vi "Write REF Channels.vi"(8 "error in (no error)":errorcluster, 10 "REF Channels":T1 {"Roll-Off" min=1; "TC" min=0.0001 format="%#_3p"; "Phase" format="%.3g"; "Frequency" min=0.0001 max=10000.0 format="%.3g"; "Channel" min=1}, 11 "DSP in":refnum<class "DSP.lvclass">) -> (0 "error out":errorcluster, 3 "DSP out":refnum<class "DSP.lvclass">)   [LabVIEW 2019, in "DSP.lvclass"]
uses:
  DSP.lvclass
  DSP.lvclass/DSP.ctl
  Typedefs/REF.Channel--Cluster.ctl
  Typedefs/REF.Channel--Cluster--Array.ctl
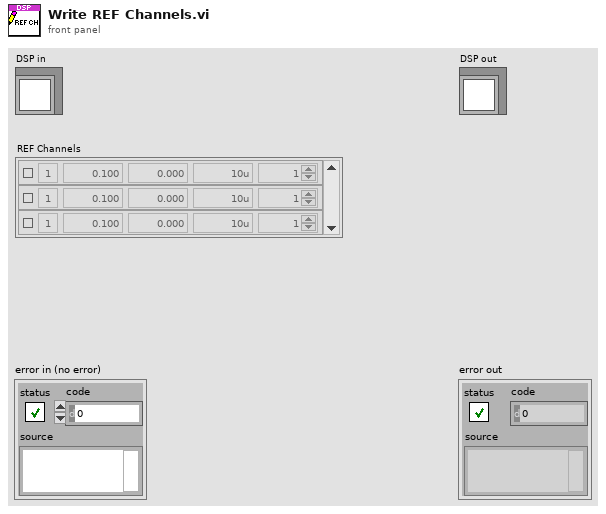
[diagram p1: front panel]
types:
  T1 = typedef "DSP.lvclass/REF.Channel--Cluster--Array.ctl" = T2[]
  T2 = typedef "DSP.lvclass/REF.Channel--Cluster.ctl" = cluster{"Enable?":bool, "Channel":i32, "Frequency":dbl, "Phase":dbl, "TC":dbl, "Roll-Off":i32}
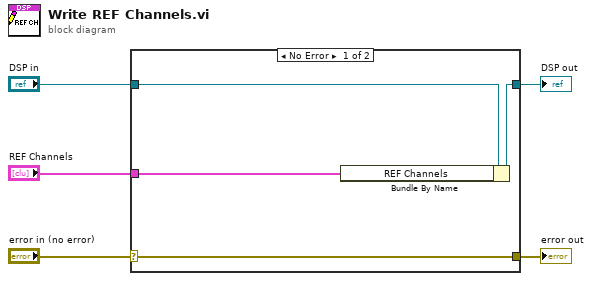
[diagram p0: block diagram]
diagram:
  n1 = case shown="No Error" "error in (no error)" {
    selector: "error in (no error)" -> [w9 w10]
    tunnel: [w9 w10] -> w4
    tunnel: [w7 w11] -> w2
    tunnel: "DSP in" -> [w8 w11]
    tunnel: "REF Channels" -> [w6 _]
    frame No Error {
      n2 = Bundle By Name(cluster=w8, "REF Channels"=w6) -> (w7:refnum<class "DSP.lvclass">)
    }
    frame Error {
    }
  }
  "error out" <- w4
  "DSP out" <- w2
